vi "VCS Set Current Regulator Gain.vi"(8 "error in (no error)":errorcluster, 10 "gains":cluster{"p-Gain":u16, "i-Gain":u16}, 11 "axis in":cluster{"keyHandle":u32, "nodeId":u16}={"keyHandle"=0, "nodeId"=1}) -> (0 "error out":errorcluster, 3 "axis out":cluster{"keyHandle":u32, "nodeId":u16}={"keyHandle"=0, "nodeId"=1})   [LabVIEW 2019, in "maxonEPOS.lvlib"]
doc: "<B>VCS Set Current Regulator Gain</B> writes all current regulator gains. Determine the optimal parameters by using the 'Regulation Tuning' of EPOS_UserInterface."
uses:
  Examples/maxonEPOS.lvlib
  Resources/EposCmd.dll
  Resources/EposCmd64.dll
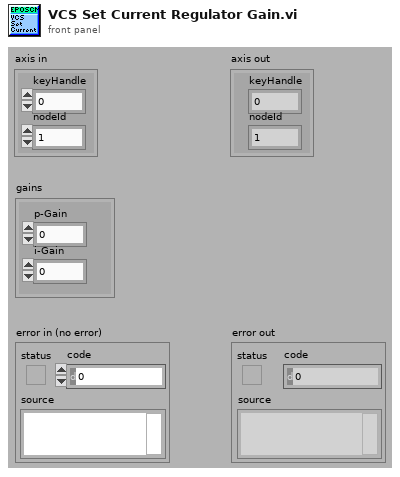
[diagram p1: front panel]
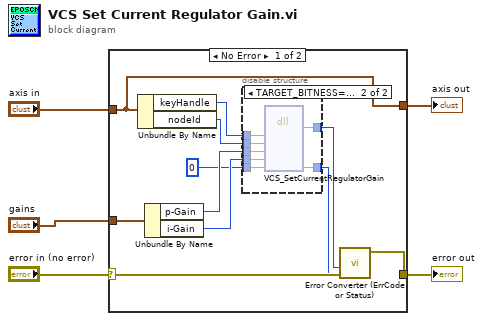
[diagram p0: block diagram]
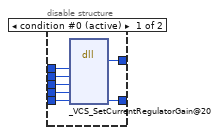
[diagram p2: hidden frame]
diagram:
  n1 = case shown="No Error" "error in (no error)" {
    selector: "error in (no error)" -> [w16 w32]
    tunnel: [w15 w32] -> w4
    tunnel: "axis in" -> [w7 w31]
    tunnel: "gains" -> [w11 _]
    tunnel: [w7 w31] -> w1
    frame No Error {
      n2 = Unbundle By Name(w7) -> ("keyHandle"=w13:u32, "nodeId"=w12:u16)
      n3 = Unbundle By Name(w11) -> ("p-Gain"=w10:u16, "i-Gain"=w9:u16)
      n4 = disable-structure shown="TARGET_BITNESS==64" {
        disable-tunnel: [w23 w30] -> w14
        disable-tunnel: w13 -> [w22 w29]
        disable-tunnel: w12 -> [w21 w28]
        disable-tunnel: w10 -> [w20 w27]
        disable-tunnel: w9 -> [w19 w26]
        disable-tunnel: u32 0 ("pErrorCode") -> [w18 w25]
        disable-tunnel: [w17 w24] -> w6
        frame condition #0 (active) {
          n5 = dll-call lib="C:/workspace/project/scancon/sw/SSI_Tool/InstrumentsInterfaces/Motordriver/maxon EPOS/Resources/EposCmd.*" fn="_VCS_SetCurrentRegulatorGain@20"("KeyHandle"=w22, "NodeId"=w21, "P"=w20, "I"=w19, "pErrorCode"=w18) -> (w17:i32, "pErrorCode"=w23:u32)  [unwired: 7 in, 2 out]
        }
        frame condition #1 {
          n6 = dll-call lib="C:/Sources/LabView/maxon EPOS/Resources/EposCmd64.*" fn="VCS_SetCurrentRegulatorGain" ("EposCmd.dll:_VCS_SetCurrentRegulatorGain@20")("KeyHandle"=w29, "NodeId"=w28, "P"=w27, "I"=w26, "pErrorCode"=w25) -> ("Rückgabetyp"=w24:i32, "pErrorCode"=w30:u32)  [unwired: 7 in, 2 out]
        }
      }
      n7 = call "Error Converter (ErrCode or Status).vi"("error code"=w14, "return type"=w6, "error in (no error)"=w16) -> ("error out"=w15:errorcluster)  [unwired: 7 in]
    }
    frame Error {
    }
  }
  "error out" <- w4
  "axis out" <- w1
